vi "Program Oscillator.vi"() -> ()   [LabVIEW 2018]
uses:
  Type/_RT Command.ctl
  <vilib>/Utility/config.llb/Read Key (U32).vi
  Configuration/_Global Configuration.vi
  <vilib>/Utility/config.llb/Write Key (Double).vi
  <vilib>/Utility/config.llb/Write Key (String).vi
  <vilib>/Utility/config.llb/Read Key (Double).vi
  <vilib>/Utility/config.llb/Write Key (U32).vi
  <vilib>/Utility/config.llb/NI_LVConfig.lvlib
panel:
  out "Frequency Tuning Word 2":u32
  out "error out":errorcluster
  in  "Read Current Osc Settings":bool caption="Note: Reference Clock is\nnot read from sbRIO"
  in  "Chip Select":u32(ring) items=["MP1-FREQ", "Q1-FREQ", "Q2-FREQ"]
  out "Register 0,1,6,7":u32=2764113333
  in  "Program":bool
  out "Frequency Tuning Word":u32
  out "Register 7":u8=181 format="%.0x"
  out "Register 6":u8=5 format="%.0x"
  out "Register 5":u8 format="%.0x"
  out "Register 4":u8 format="%.0x"
  out "Register 3":u8 format="%.0x"
  out "Register 2":u8=64 format="%.0x"
  out "Register 1":u8=193 format="%.0x"
  out "Register 0":u8=164 format="%.0x"
  in  "Amplitude Scale Factor":dbl=0.6 min=0.0 max=1.9921875 format="%#.1g"
  in  "Frequency Out (MHz)":dbl=1.0 min=0.0 max=1000.0 format="%#.2g"
  in  "Reference Clock Multiplier":dbl=10.0 min=4.0 max=20.0 step=1.0 format="%#.8g"
  in  "Reference Clock (MHz)":dbl=10.0 min=0.0 max=1000.0 format="%#.8g"
  # "Warning: The values below do not necessary represent the current instrument settings."
  # "(160 + the Reference Clock Multipler value)"
  # "(193, the value to select single tone mode, DPD pin for shutdown, no SLEEP mode)"
  # "(the 1st 8 bits of the frequency tuning word)"
  # "(the 2nd 8 bits of the frequency tuning word)"
  # "(the 3rd 8 bits of the frequency tuning word)"
  # "(the last 8 bits of the frequency tuning word)"
  # "(5, the value to bypass the CIC filter)"
  # "(128 * the Amplitude Scale Factor)"
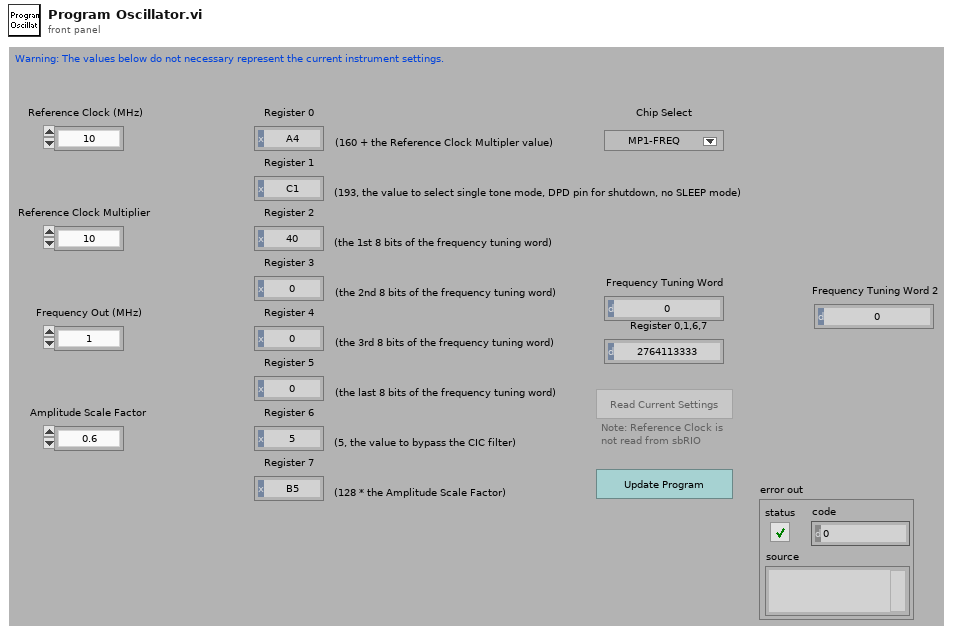
[diagram p1: front panel]
types:
  T1 = enum8{"Enabled", "Disabled", "Disabled and Grayed Out"}
  T2 = typedef "_RT Command.ctl" = enum16{"xml Start Run", "xml Start Actual Run", "xml Stop Run", "xml Runtime Update", "xml Get Status", "xml Get Table", "xml Set Table", "xml Get Configuration", "xml System Status", "xml Set LC Input Logic", "xml Get Data", "xml Get Info", "Start", "StartActualRun", "Stop", "Runtime Update", "Get Data", "Get Info", "Get Status", "Get Param", "Get Config", "Get Table", "Read ADC", "Set Oscillator", "Update Config", "Update Table", "Set All Pol", "Set Pol and DC", "Set Max Mass", "Toggle RP", "Toggle EL", "Set PIC", "Initialize Turbo", "Send Turbo Comm", "Close Turbo", "P1", "P2", "P3", "Send Serial", "Set LC Out", "Get LC In", "Read VAC", "Test Table", "Toggle Power", "Get Startup", "Set Startup", "Get ADC Table", "Set ADC Table", "Get Brief Status", "Get Detail Status", "Auxiliary Update", "Set CC Logics", "Set CC Input Logics", "Ignore Error", "invalid"}
  T3 = typedef "NI_LVConfig.lvlib/Config Data RefNum.ctl" = refnum<k1>
  T4 = typedef "_RT Instrument 2.ctl" = cluster{"Table":T5[], "Instrument":string[]}
  T5 = typedef "_RT Configuration 2.ctl" = cluster{"Name":string, "Ch#":u8, "Min":dbl, "Max":dbl, "Def+":dbl, "Def-":dbl, "Offset":dbl, "Slope":dbl, "Type":u8, "Description":string, "SettleT":dbl}
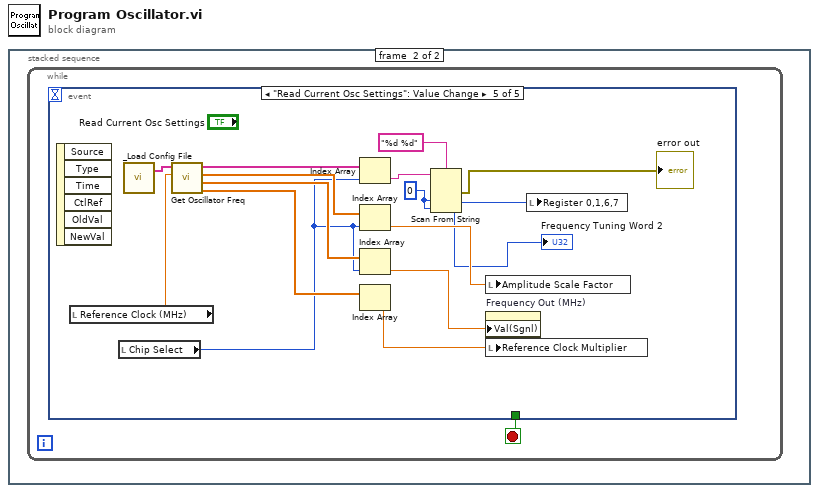
[diagram p0: block diagram]
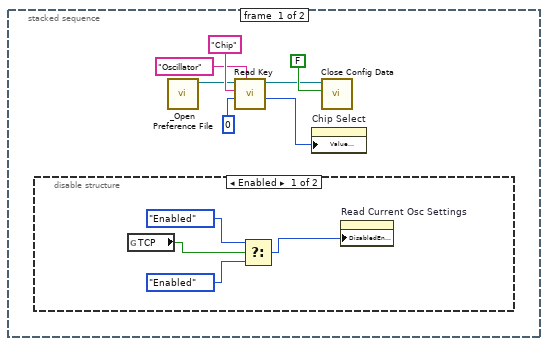
[diagram p2: hidden frame]
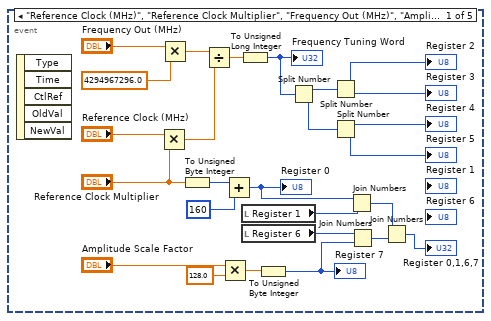
[diagram p4: hidden frame]
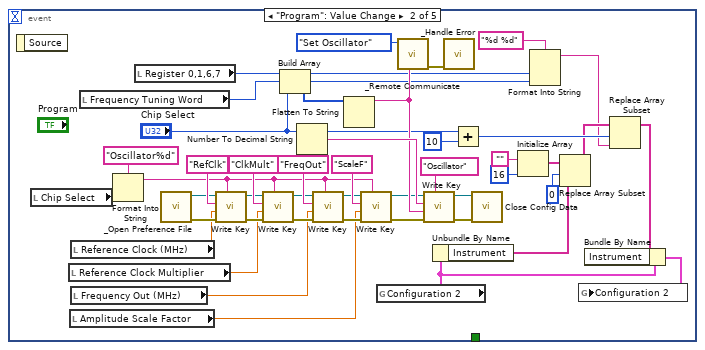
[diagram p5: hidden frame]
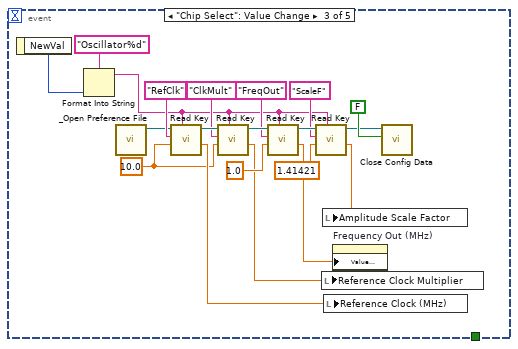
[diagram p6: hidden frame]
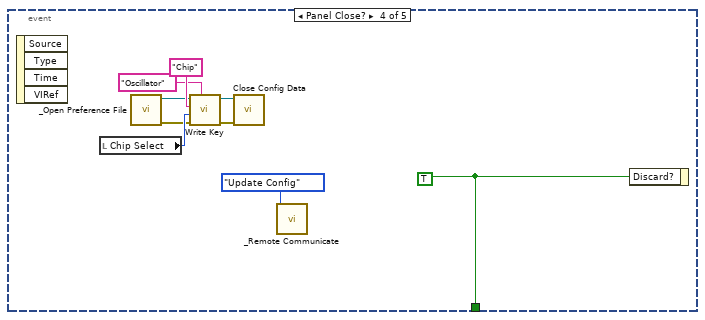
[diagram p7: hidden frame]
diagram:
  n1 = stacked-sequence {
    frame #0 {
      n2 = disable-structure shown="Enabled" {
        frame Enabled {
          n3 = global read "_Global Configuration.vi" "TCP"() -> (w9:bool)
          n4 = Select(t=T1."Enabled" ("Disabled"), s=w9, f=T1."Enabled" ("Disabled")) -> (s? t:f=w8:T1)
          n5 = property on="Read Current Osc Settings" class="Bool"("DisabledEnum"=w8) -> ()  [unwired: 2 in, 2 out]
        }
        frame Disabled {
        }
      }
      n6 = call "_Open Preference File.vi"() -> ("refnum"=w2:T3)  [unwired: 3 in, 4 out]
      n7 = call-poly <vilib>:"Read Key.vi"("section"="Oscillator", "default value"=u32 0 ("Chip Select"), "key"="Chip" ("section"), "refnum"=w2) -> ("value"=w3:u32, "refnum out"=w5:T3)  [unwired: 1 in, 5 out]
      n8 = property on="Chip Select" class="Ring (strict)"("Value (Signaling)"=w3) -> ()  [unwired: 2 in, 2 out]
      n9 = call <vilib>:"Close Config Data.vi"("write file if changed (T)"=FALSE ("write configuration file? (T)"), "refnum"=w5) -> ()  [unwired: 1 in, 9 out]
    }
    frame #1 {
      n10 = while {
        stop <- w12 stop-if-true
        n11 = event shown="[4] \"Read Current Osc Settings\": Value Change" {
          selector: _ -> [_ _ _ _ _]
          dyn-events: _ -> [_ _ _ _ _]
          timeout: _ -> [_ _ _ _ _]
          tunnel: [_ _ _ w112 _] -> w12
          event "Reference Clock (MHz)", "Reference Clock Multiplier", "Frequency Out (MHz)", "Amplitude Scale Factor": Value Change {
            n12 = event-data() -> ()  [unwired: 6 out]
            n13 = Multiply(x="Reference Clock (MHz)", y="Reference Clock Multiplier") -> (x*y=w34:dbl)
            n14 = Multiply(x="Frequency Out (MHz)", y=4294967296.0) -> (x*y=w35:dbl)
            n15 = To Unsigned Byte Integer(number="Reference Clock Multiplier") -> (unsigned 8bit integer=w23:u8)
            n16 = Divide(x=w35, y=w34) -> (x/y=w33:dbl)
            n17 = Multiply(x="Amplitude Scale Factor", y=128.0) -> (x*y=w22:dbl)
            n18 = Add(x=w23, y=u8 160) -> (x+y=w19:u8)
            "Register 0" <- w19
            n19 = To Unsigned Long Integer(number=w33) -> (unsigned 32bit integer=w32:u32)
            "Frequency Tuning Word" <- w32
            n20 = local read "Register 1"() -> (w18:u8)
            n21 = local read "Register 6"() -> (w15:u8)
            n22 = To Unsigned Byte Integer(number=w22) -> (unsigned 8bit integer=w13:u8)
            "Register 7" <- w13
            n23 = Split Number(x=w32) -> (hi(x)=w31:u16, lo(x)=w30:u16)
            n24 = Split Number(x=w31) -> (hi(x)=→"Register 2":u8, lo(x)=→"Register 3":u8)
            n25 = Split Number(x=w30) -> (hi(x)=→"Register 4":u8, lo(x)=→"Register 5":u8)
            n26 = Join Numbers(hi=w19, lo=w18) -> ((hi.lo)=w17:u16)
            n27 = Join Numbers(hi=w15, lo=w13) -> ((hi.lo)=w16:u16)
            n28 = Join Numbers(hi=w17, lo=w16) -> ((hi.lo)=→"Register 0,1,6,7":u32)
          }
          event "Program": Value Change {
            n29 = event-data() -> ()  [unwired: 2 out]
            n30 = local read "Chip Select"() -> (w56:u32)
            n31 = local read "Reference Clock Multiplier"() -> (w62:dbl)
            n32 = local read "Amplitude Scale Factor"() -> (w60:dbl)
            n33 = local read "Reference Clock (MHz)"() -> (w63:dbl)
            n34 = local read "Frequency Out (MHz)"() -> (w61:dbl)
            n35 = local read "Frequency Tuning Word"() -> (w52:u32)
            n36 = Format Into String(format string="Oscillator%d", w56) -> (resulting string=w55:string)  [unwired: 2 in, 1 out]
            n37 = local read "Register 0,1,6,7"() -> (w53:u32)
            n38 = call "_Open Preference File.vi"() -> ("error"=w72:errorcluster, "refnum"=w67:T3)  [unwired: 3 in, 3 out]
            n39 = call-poly <vilib>:"Write Key.vi"("section"=w55, "error in (no error)"=w72, "value"=w63, "key"="RefClk" ("section"), "refnum"=w67) -> ("error out"=w73:errorcluster, "refnum out"=w66:T3)  [unwired: 3 in, 2 out]
            n40 = call-poly <vilib>:"Write Key.vi"("section"=w55, "error in (no error)"=w73, "value"=w62, "key"="ClkMult" ("section"), "refnum"=w66) -> ("error out"=w74:errorcluster, "refnum out"=w65:T3)  [unwired: 3 in, 2 out]
            n41 = Build Array(w53, w52, "Chip Select") -> (w83:u32[])
            n42 = Number To Decimal String(number="Chip Select") -> (decimal integer string=w79:string)  [unwired: 1 out]
            n43 = call-poly <vilib>:"Write Key.vi"("section"=w55, "error in (no error)"=w74, "value"=w61, "key"="FreqOut" ("section"), "refnum"=w65) -> ("error out"=w75:errorcluster, "refnum out"=w64:T3)  [unwired: 3 in, 2 out]
            n44 = Flatten To String(anything=w83) -> (data string=w78:string)  [unwired: 1 in, 4 out]
            n45 = call-poly <vilib>:"Write Key.vi"("section"=w55, "error in (no error)"=w75, "value"=w60, "key"="ScaleF" ("section"), "refnum"=w64) -> ("error out"=w58:errorcluster, "refnum out"=w59:T3)  [unwired: 3 in, 2 out]
            n46 = global read "_Global Configuration.vi" "Configuration 2"() -> (w54:T4)
            n47 = call "_Remote Communicate.vi"("String"=w78, "Command"=_RT_Command."Set Oscillator") -> ("error out"=w81:errorcluster)  [unwired: 4 in, 3 out]
            n48 = call-poly <vilib>:"Write Key.vi"("section"="Oscillator", "error in (no error)"=w58, "value"=w78, "key"=w79, "refnum"=w59) -> ("error out"=w76:errorcluster, "refnum out"=w77:T3)  [unwired: 1 in, 4 out]
            n49 = Unbundle By Name(w54) -> ("Instrument"=w43:string[])
            n50 = call "_Handle Error.vi"("error in (no error)"=w81) -> ()  [unwired: 2 in, 5 out]
            n51 = Add(x="Chip Select", y=u32 10) -> (x+y=w46:u32)
            n52 = call <vilib>:"Close Config Data.vi"("error in (no error)"=w76, "refnum"=w77) -> ()  [unwired: 1 in, 9 out]
            n53 = Initialize Array("", 16 ("dimension size")) -> (w45:string[])
            n54 = Format Into String(format string="%d %d", w53, w52) -> (resulting string=w41:string)  [unwired: 2 in, 1 out]
            n55 = Replace Array Subset(array=w45, new element=w43, index=0) -> (w42:string[])
            n56 = Replace Array Subset(array=w42, new element=w41, index=w46) -> (w40:string[])
            n57 = Bundle By Name(cluster=w54, "Instrument"=w40) -> (w39:T4)
            n58 = global write "_Global Configuration.vi" "Configuration 2"(w39) -> ()
          }
          event "Chip Select": Value Change {
            w84 = 10.0 ("Value (Signaling)")
            n59 = event-data() -> ("NewVal"=w88:u32)  [unwired: 1 out]
            n60 = Format Into String(format string="Oscillator%d", w88) -> (resulting string=w86:string)  [unwired: 2 in, 1 out]
            n61 = call "_Open Preference File.vi"() -> ("refnum"=w102:T3)  [unwired: 3 in, 4 out]
            n62 = call-poly <vilib>:"Read Key.vi"("section"=w86, "default value"=w84, "key"="RefClk" ("section"), "refnum"=w102) -> ("value"=w91:dbl, "refnum out"=w101:T3)  [unwired: 1 in, 5 out]
            n63 = call-poly <vilib>:"Read Key.vi"("section"=w86, "default value"=w84, "key"="ClkMult" ("section"), "refnum"=w101) -> ("value"=w92:dbl, "refnum out"=w100:T3)  [unwired: 1 in, 5 out]
            n64 = call-poly <vilib>:"Read Key.vi"("section"=w86, "default value"=1.0 ("Value (Signaling)"), "key"="FreqOut" ("section"), "refnum"=w100) -> ("value"=w93:dbl, "refnum out"=w99:T3)  [unwired: 1 in, 5 out]
            n65 = call-poly <vilib>:"Read Key.vi"("section"=w86, "default value"=1.41421 ("Value (Signaling)"), "key"="ScaleF" ("section"), "refnum"=w99) -> ("value"=w89:dbl, "refnum out"=w85:T3)  [unwired: 1 in, 5 out]
            n66 = local write "Reference Clock Multiplier"(w92) -> ()
            n67 = local write "Amplitude Scale Factor"(w89) -> ()
            n68 = local write "Reference Clock (MHz)"(w91) -> ()
            n69 = property on="Frequency Out (MHz)" class="DigNum (strict)"("Value (Signaling)"=w93) -> ()  [unwired: 2 in, 2 out]
            n70 = call <vilib>:"Close Config Data.vi"("write file if changed (T)"=FALSE ("write configuration file? (T)"), "refnum"=w85) -> ()  [unwired: 1 in, 9 out]
          }
          event Panel Close? {
            w112 = TRUE
            n71 = event-data() -> ()  [unwired: 5 out]
            n72 = local read "Chip Select"() -> (w108:u32)
            n73 = call "_Open Preference File.vi"() -> ("error"=w105:errorcluster, "refnum"=w106:T3)  [unwired: 3 in, 3 out]
            n74 = call-poly <vilib>:"Write Key.vi"("section"="Oscillator", "error in (no error)"=w105, "value"=w108, "key"="Chip" ("section"), "refnum"=w106) -> ("error out"=w110:errorcluster, "refnum out"=w109:T3)  [unwired: 5 out]
            n75 = call <vilib>:"Close Config Data.vi"("error in (no error)"=w110, "refnum"=w109) -> ()  [unwired: 1 in, 9 out]
            n76 = call "_Remote Communicate.vi"("Command"=_RT_Command."Update Config") -> ()  [unwired: 5 in, 4 out]
            n77 = event-data("Discard?"=w112) -> ()  [unwired: 1 in, 1 out]
          }
          event "Read Current Osc Settings": Value Change {
            w124 = u32 0 ("Frequency Tuning Word")
            n78 = event-data() -> ()  [unwired: 7 out]
            n79 = local read "Reference Clock (MHz)"() -> (w116:dbl)
            n80 = local read "Chip Select"() -> (w115:u32)
            n81 = call "_Load Config File.vi"() -> ("Instrument"=w128:string[])  [unwired: 2 in, 1 out]
            n82 = call "Get Oscillator Freq.vi"("Reference Clock"=w116, "Array 3"=w128) -> ("Reference Clock Multiplier"=w119:dbl[], "Oscillator Freqs"=w121:dbl[], "Scaling Factor"=w122:dbl[], "Tuning Word"=w127:string[])  [unwired: 6 in]
            n83 = Index Array(array=w127, index=w115) -> (element=w126:string)
            n84 = Index Array(array=w122, index=w115) -> (element=w120:dbl)
            n85 = Index Array(array=w121, index=w115) -> (element=w118:dbl)
            n86 = Index Array(array=w119) -> (element=w117:dbl)  [unwired: 1 in]
            n87 = Scan From String(format string="%d %d", input string=w126, default 1=w124, default 2=w124) -> (error out=→"error out":errorcluster, output 1=w123:u32, output 2=→"Frequency Tuning Word 2":u32)  [unwired: 2 in, 2 out]
            n88 = local write "Amplitude Scale Factor"(w120) -> ()
            n89 = property on="Frequency Out (MHz)" class="DigNum (strict)"("Val(Sgnl)"=w118) -> ()  [unwired: 2 in, 2 out]
            n90 = local write "Reference Clock Multiplier"(w117) -> ()
            n91 = local write "Register 0,1,6,7"(w123) -> ()
          }
        }
      }
    }
  }
